vi "Vision Research Phantom Series PhFile PhGetWriteCineFileProgressAll.vi"(1 "pCount [in]":u32, 5 "Error In (no error)":errorcluster) -> (14 "pSaveCineInfo [out]":i32, 15 "pCount [out]":u32, 19 "Error Out":errorcluster)   [LabVIEW 2013, in "VRI.lvlib"]
doc: "PhGetWriteCineFileProgressAll\nHRESULT PhGetWriteCineFileProgressAll(PSAVECINEINFO pSaveCineInfo, PUINT pCount);\n\nParameters\npSaveCineInfo [out]\n Preallocated array of SAVECINEINFO elements to be filled with information about all currently active write cine file operations.\npCount [in, out]\n Input: pSaveCineInfo size.\n Output: number of filled elements in pSaveCineInfo array.\n\nReturn Value\nThe function returns ERR_Ok in case of success or an error code, otherwise. To get extended error information call PhGetErrorMessage.\n\nRemarks\nReturns progress information about all synchronous and asynchronous currently active write cine file operations.\n\nRequired Header\nPhFile.h"
uses:
  VRI.lvlib
  Phantom DLLs/PhFile.Dll
panel:
  # "For instructions on the use of this VI, press Ctrl+H to display the help window and move the mouse over the icon, controls, and indicators"
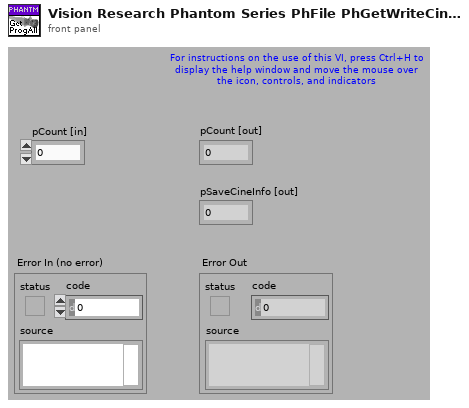
[diagram p1: front panel]
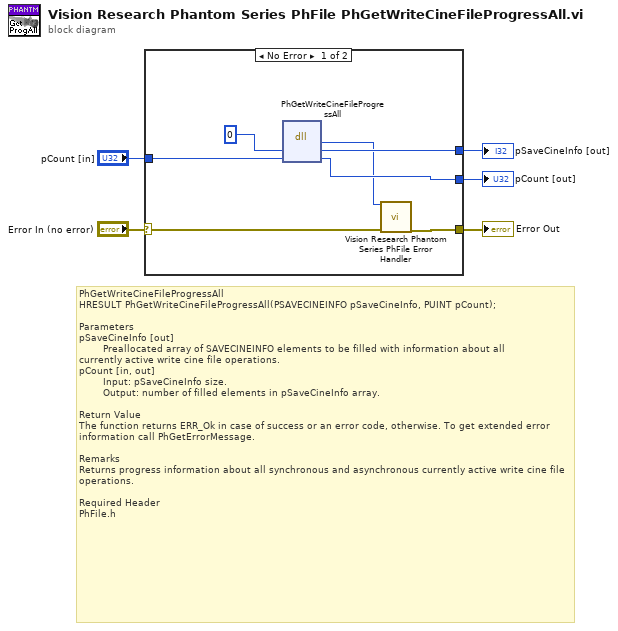
[diagram p0: block diagram]
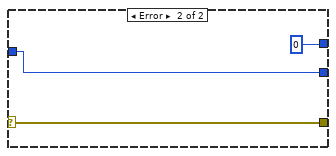
[diagram p2: hidden frame]
diagram:
  # "PhGetWriteCineFileProgressAll\nHRESULT PhGetWriteCineFileProgressAll(PSAVECINEINFO pSaveCineInfo, PUINT pCount);\n\nParameters\npSaveCineInfo [out]\n        Preallocated array of SAVECINEINFO elements to be filled with information about all                                            currently active write cine file operations.\npCount [in, out]\n\t       Input: pSaveCineInfo size.\n\t       Output: number of filled elements in pSaveCineInfo array.\n\nReturn Value\nThe function returns ERR_Ok in case of success or an error code, otherwise. To get extended error information call PhGetErrorMessage.\n\nRemarks\nReturns progress information about all synchronous and asynchronous currently active write cine file operations.\n\nRequired Header\nPhFile.h"
  n1 = case shown="No Error" "Error In (no error)" {
    selector: "Error In (no error)" -> [w12 w15]
    tunnel: [w11 w15] -> w4
    tunnel: "pCount [in]" -> [w10 w14]
    tunnel: [w9 0] -> w2
    tunnel: [w8 w14] -> w1
    frame No Error {
      n2 = dll-call lib="C:/Projects/SDK/64-bit/Vision Research Phantom Series Labview Driver/Phantom DLLs/PhFile.dll" fn="PhGetWriteCineFileProgressAll"("pSaveCineInfo"=0, "pCount"=w10) -> ("HRESULT"=w6:i32, "pSaveCineInfo"=w9:i32, "pCount"=w8:u32)  [unwired: 3 in, 2 out]
      n3 = call "Vision Research Phantom Series PhFile Error Handler.vi"("Error Code (0)"=w6, "Error In (no error)"=w12) -> ("Error Out"=w11:errorcluster)  [unwired: 17 out]
    }
    frame Error {
    }
  }
  "Error Out" <- w4
  "pSaveCineInfo [out]" <- w2
  "pCount [out]" <- w1
